vi "HW2-j&j.vi"(9 "AM Wave Parameters":T1, 10 "Digitizing Parameters":T2) -> (2 "AM Wave":cluster{"Time":dbl[], "Displacement":dbl[]})   [LabVIEW 2015]
uses:
  <vilib>/imath/engines/lvmath2/RunTimeEngine/Managers/WorkSpace/UID Generator.vi
  <vilib>/imath/engines/lvmath2/RunTimeEngine/RunTimeType/NIMS_RunTimeType_From StrictType (excl LVString).vi
  <instcachedir>/0/NIMS_RunTimeType_From StrictType (excl LVString)_EB1C38A9BC5048DA9ABDA8F781E54D21.lvgen/NIMS_RunTimeType_From StrictType (excl LVString)_EB1C38A9BC5048DA9ABDA8F781E54D21_000.vi
  <vilib>/imath/engines/lvmath2/RunTimeEngine/LocalVariableDefStatement/MC_LocalVariableDefStatement_Display.vi
  <vilib>/imath/engines/lvmath2/RunTimeEngine/RangeToken/NIMS_Range.vi
  <instcachedir>/0/NIMS_Range_D919CC09935940E88F755EC1C6F49AC1.lvgen/NIMS_Range_D919CC09935940E88F755EC1C6F49AC1_000.vi
  <vilib>/imathl/engines/lvmath/Functions/Error Handling/Create Error.vi
  <vilib>/imath/engines/lvmath2/RunTimeEngine/ArithmeticOperatorToken/NIMS_ArithmeticOperator_times.vi
  <instcachedir>/0/NIMS_ArithmeticOperator_times_DF26C4080E2A467BA28C929B8CF31953.lvgen/NIMS_ArithmeticOperator_times_DF26C4080E2A467BA28C929B8CF31953_000.vi
  <vilib>/imath/engines/lvmath2/RunTimeEngine/BuiltInFunctions/gensignal/NIMS_gensignal(str,RS,RS,RS).vi
  <vilib>/imath/engines/lvmath2/RunTimeEngine/BuiltInFunctions/transpose/NIMS_transpose(GV).vi
  <instcachedir>/0/NIMS_transpose(GV)_1D76875BF542458FA31D2D0CC3E998C0.lvgen/NIMS_transpose(GV)_1D76875BF542458FA31D2D0CC3E998C0_000.vi
  <vilib>/imath/engines/lvmath2/RunTimeEngine/BuiltInFunctions/linramp/NIMS_linramp.vi
  <vilib>/imath/engines/lvmath2/RunTimeEngine/VariableToken/NIMS_VariableToken_CondDefined.vi
  <instcachedir>/0/NIMS_VariableToken_CondDefined_FE30D0A1BFB24F098D41DEBABFE96BE1.lvgen/NIMS_VariableToken_CondDefined_FE30D0A1BFB24F098D41DEBABFE96BE1_003.vi
  <vilib>/imath/engines/lvmath/Functions/Error Handling/MergeErrorsWrapper.vi
  <vilib>/imath/engines/lvmath2/RunTimeEngine/Managers/SymbolTable/Clear UID.vi
  <vilib>/imath/engines/lvmath2/RunTimeEngine/NodeEndStatement/NIMS_NodeEndStatement_Output.vi
  <instcachedir>/0/NIMS_NodeEndStatement_Output_53EC0D466D134D7ABD903AC30B43404B.lvgen/NIMS_NodeEndStatement_Output_53EC0D466D134D7ABD903AC30B43404B_005.vi
  <vilib>/imath/engines/lvmath2/RunTimeEngine/ErrorHandling/NIMS_Finalize Error.vi
  <vilib>/imath/engines/lvmath2/RunTimeEngine/Managers/SymbolTable/NIMS_WorkSpace.lvlib
panel:
  out "XY Graph":cluster{"t":dbl[], "x":dbl[]}(graph)
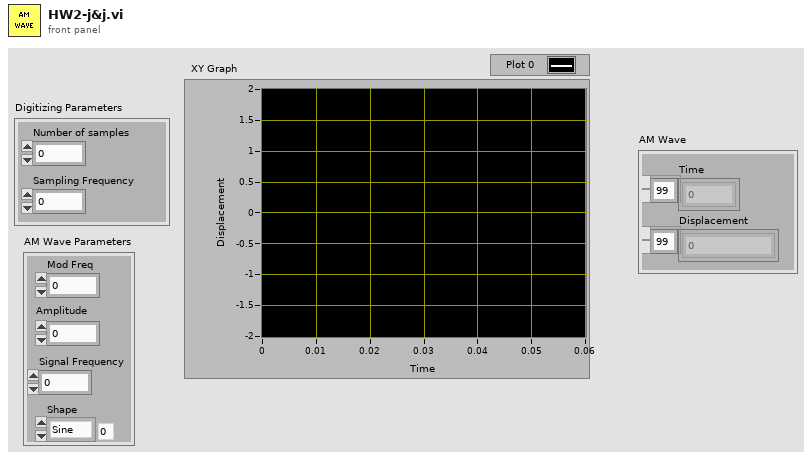
[diagram p1: front panel]
types:
  T1 = cluster{"Mod Freq":dbl, "Amplitude":dbl, "Shape":enum16{"Sine", "Cosine", "DC Level", "Square", "User Defined"}, "Signal Frequency":dbl}
  T2 = cluster{"Number of samples":dbl, "Sampling Frequency":dbl}
  T3 = enum16{"Sine", "Cosine", "DC Level", "Square", "User Defined"}
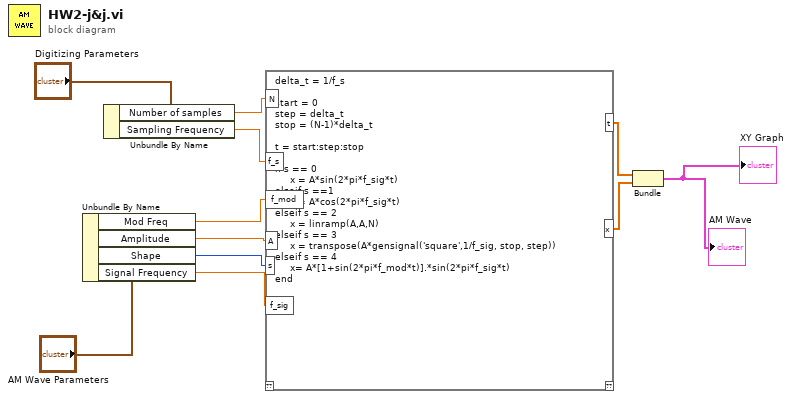
[diagram p0: block diagram]
diagram:
  n1 = Unbundle By Name("AM Wave Parameters") -> ("Mod Freq"=w5:dbl, "Amplitude"=w4:dbl, "Shape"=w3:T3, "Signal Frequency"=w1:dbl)
  n2 = Unbundle By Name("Digitizing Parameters") -> ("Number of samples"=w8:dbl, "Sampling Frequency"=w7:dbl)
  n3 = mathscript code="delta_t = 1/f_s\n\nstart = 0\nstep = delta_t\nstop = (N-1)*delta_t\n\nt = start:step:stop\n\nif s == 0\n     x = A*sin(2*pi*f_sig*t)\nelseif s ==1\n     x = A*cos(2*pi*f_sig*t)   \nelseif s == 2\n     x = linramp(A,A,N)\nelseif s == 3\n     x = transpose(A*gensignal('square',1/f_sig, stop, step))\nelseif s == 4\n     x= A*[1+sin(2*pi*f_mod*t)].*sin(2*pi*f_sig*t)\nend"("N"=w8, "f_s"=w7, "f_mod"=w5, "A"=w4, "s"=w3, "f_sig"=w1) -> ("x"=w11:dbl[], "t"=w10:dbl[])  [unwired: 1 in, 1 out]
  n4 = Bundle("t"=w10, "x"=w11) -> (→"XY Graph" →"AM Wave":cluster{"t":dbl[], "x":dbl[]})  [unwired: 1 in]
